vi "HardwareStop.vi"(8 "Error In":errorcluster, 11 "Keithley 7001 In":refnum<visa-resource-name>) -> (0 "Error Out":errorcluster, 3 "Keithley 7001 Out":refnum<visa-resource-name>)   [LabVIEW 2012]
uses:
  driver/Public/Controls/Slot.ctl
  driver/Keithley-7001.lvlib
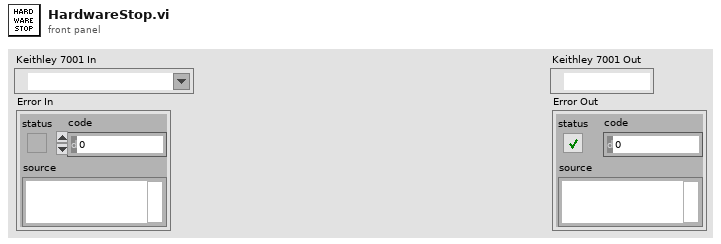
[diagram p1: front panel]
types:
  T1 = typedef "Keithley-7001.lvlib/Slot.ctl" = enum16{"Slot 1", "Slot 2"}
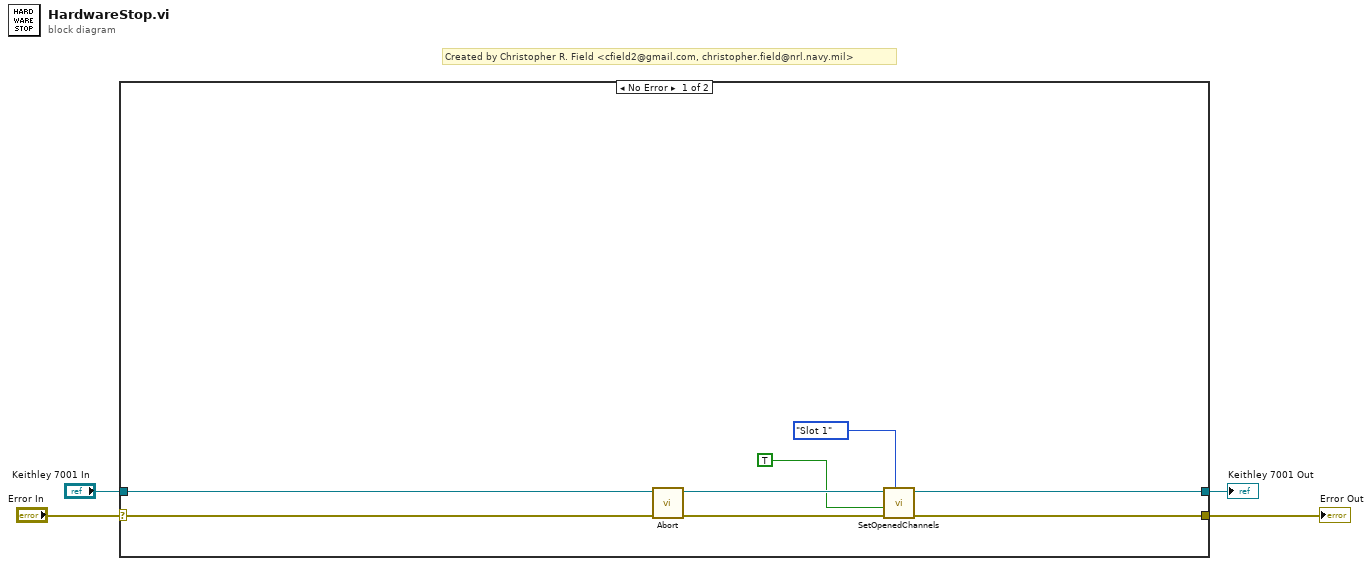
[diagram p0: block diagram]
diagram:
  # "Created by Christopher R. Field <cfield2@gmail.com, christopher.field@nrl.navy.mil>"
  n1 = case shown="No Error" "Error In" {
    selector: "Error In" -> [w11 w13]
    tunnel: "Keithley 7001 In" -> [w12 w14]
    tunnel: [w8 w13] -> w1
    tunnel: [w7 w14] -> w2
    frame No Error {
      n2 = call "Abort.vi"("Error In"=w11, "Keithley 7001 In"=w12) -> ("Error Out"=w9:errorcluster, "Keithley 7001 Out"=w10:refnum<visa-resource-name>)  [unwired: 8 in]
      n3 = call "SetOpenedChannels.vi"("Slot"=Slot."Slot 1", "Error In"=w9, "All?"=TRUE, "Keithley 7001 In"=w10) -> ("Error Out"=w8:errorcluster, "Keithley 7001 Out"=w7:refnum<visa-resource-name>)  [unwired: 6 in]
    }
    frame Error {
    }
  }
  "Keithley 7001 Out" <- w2
  "Error Out" <- w1
